vi "Fit.vi"(7 "Type X":T1(ring), 8 "error in (no error)":errorcluster caption="entrée d'erreur (pas d'erreur)", 9 "y":string[][](array[string]), 10 "X":string[][](array[string]), 11 "SimpleImputer.lvclass":refnum<class "SimpleImputer.lvclass">) -> (0 "error out":errorcluster caption="sortie d'erreur", 2 "String Data":string, 3 "SimpleImputer.lvclass":refnum<class "SimpleImputer.lvclass">)   [LabVIEW 2020, in "SimpleImputer.lvclass"]
doc: "Fit the imputer on X.\n\nReturns : \n\n- String : OK"
uses:
  SimpleImputer.lvclass
  SimpleImputer.lvclass/SimpleImputer.ctl
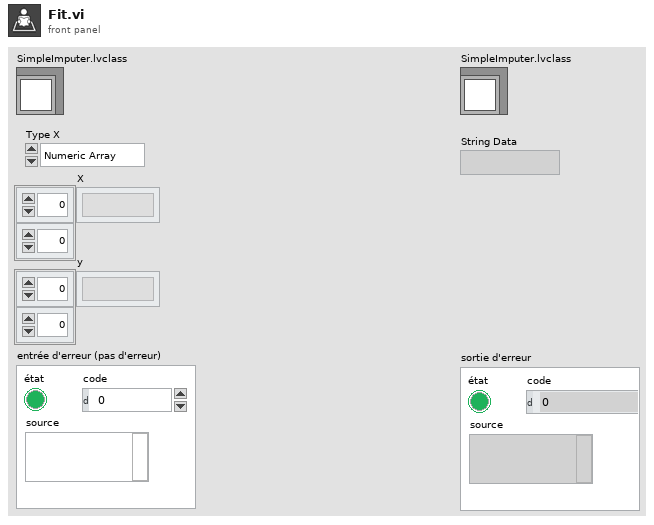
[diagram p1: front panel]
types:
  T1 = enum16{"Numeric Array", "String Array", "Sparse"}
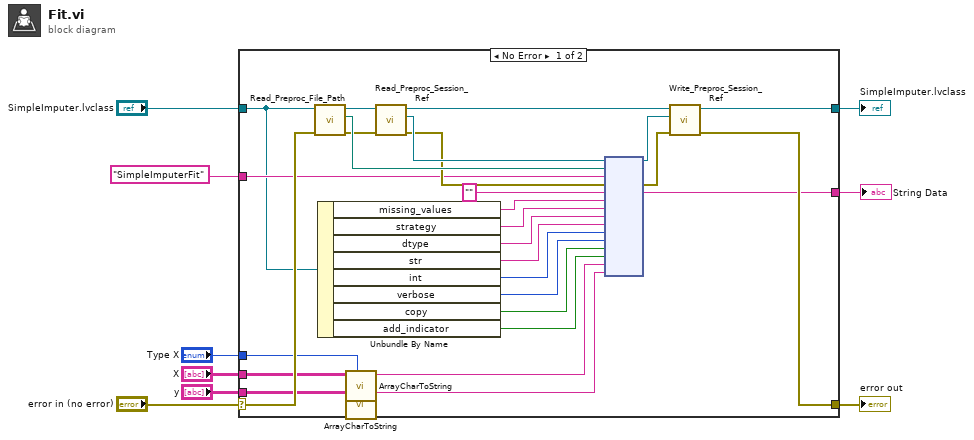
[diagram p0: block diagram]
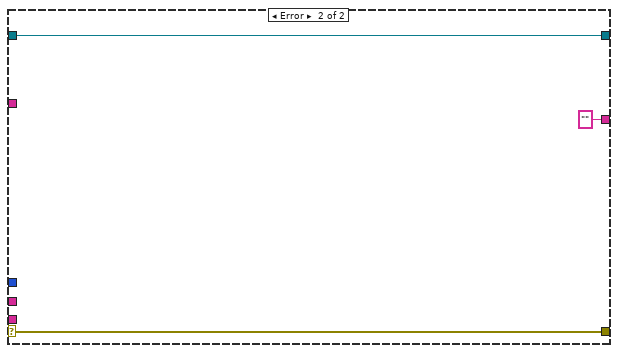
[diagram p2: hidden frame]
diagram:
  n1 = case shown="No Error" "error in (no error)" {
    selector: "error in (no error)" -> [w28 w40]
    tunnel: [w27 w40] -> w8
    tunnel: [w26 w39] -> w6
    tunnel: "SimpleImputer.lvclass" -> [w23 w39]
    tunnel: "SimpleImputerFit" ("Fonction") -> [w25 _]
    tunnel: [w24 ""] -> w4
    tunnel: "X" -> [w14 _]
    tunnel: "y" -> [w11 _]
    tunnel: "Type X" -> [w12 _]
    frame No Error {
      n2 = call-dynamic "Read_Preproc_File_Path.vi"("error in (no error)"=w28, "Python in"=w23) -> ("error out"=w32:errorcluster, "File_Path"=w35:path, "Python out"=w37:refnum<class "SimpleImputer.lvclass">)  [unwired: 7 in]
      n3 = Unbundle By Name(w23) -> ("missing_values"=w22:string, "strategy"=w21:string, "dtype"=w20:string, "str"=w19:string, "int"=w18:i32, "verbose"=w17:i32, "copy"=w16:bool, "add_indicator"=w15:bool)
      n4 = call "ArrayCharToString.vi"("Type"=w12, "TAB"=w14) -> ("Instruction"=w13:string)  [unwired: 9 in]
      n5 = call "ArrayCharToString.vi"("TAB"=w11) -> ("Instruction"=w10:string)  [unwired: 10 in]
      n6 = call-dynamic "Read_Preproc_Session_Ref.vi"("error in (no error)"=w32, "Python in"=w37) -> ("error out"=w33:errorcluster, "Session_ref"=w34:refnum<k35>, "Python out"=w36:refnum<class "SimpleImputer.lvclass">)  [unwired: 7 in]
      n7 = node(w34, w35, w25, w33, "", w22, w21, w20, w19, w18, w17, w16, w15, w13, w10) -> (w29:refnum<k35>, w31:errorcluster, w24:string)  [unwired: 10 in, 2 out]
      n8 = call-dynamic "Write_Preproc_Session_Ref.vi"("error in (no error)"=w31, "Session_ref"=w29, "Python in"=w36) -> ("error out"=w27:errorcluster, "Python out"=w26:refnum<class "SimpleImputer.lvclass">)  [unwired: 7 in]
    }
    frame Error {
    }
  }
  "error out" <- w8
  "SimpleImputer.lvclass" <- w6
  "String Data" <- w4
